vi "Set XY Voltage.vi"(1 "Y-Position":dbl, 2 "X-Position":dbl) -> ()   [LabVIEW 2014]
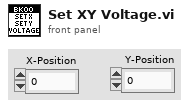
[diagram p1: front panel]
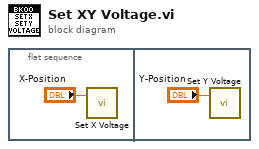
[diagram p0: block diagram]
diagram:
  n1 = flat-sequence {
    frame #0 {
      n2 = call "Set X Voltage.vi"("X position (V)"="X-Position") -> ()  [unwired: 2 in]
    }
    frame #1 {
      n3 = call "Set Y Voltage.vi"("Y position (V)"="Y-Position") -> ()  [unwired: 2 in]
    }
  }
